vi "Open Gyro.vi"(8 "Gain":dbl=0.07, 9 "Analog Channel":T1=enum."AI 1", 11 "Gyro ID (1 or 2)":i32) -> ()   [LabVIEW 2015]
uses:
  <vilib>/Rock Robotics/SystemInterfaces/AI/FPGA_AIChannel.ctl
  Robot Global Data.vi
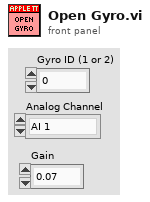
[diagram p1: front panel]
types:
  T1 = typedef "FPGA_AIChannel.ctl" = enum8{"AI 0", "AI 1", "AI 2", "AI 3", "AI MXP 0", "AI MXP 1", "AI MXP 2", "AI MXP 3", "Invalid"}
  T2 = typedef "WPI_AnalogChannelDevRef.ctl" = cluster{"DevStatus":errorcluster, "Analog Channel":T1}
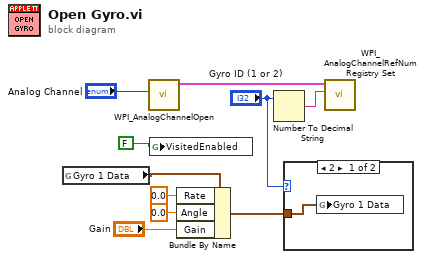
[diagram p0: block diagram]
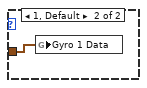
[diagram p2: hidden frame]
diagram:
  n1 = global read "Robot Global Data.vi" "Gyro 1 Data"() -> (w2:cluster{"Rate":dbl, "Angle":dbl, "Gain":dbl})
  n2 = call <vilib>:"WPI_AnalogChannelOpen.vi"("Analog Channel"="Analog Channel") -> ("AIDeviceRef"=w9:T2)  [unwired: 9 in, 1 out]
  n3 = global write "Robot Global Data.vi" "VisitedEnabled"(FALSE ("VisitedEnabled")) -> ()
  n4 = Bundle By Name(cluster=w2, "Rate"=0.0, "Angle"=0.0, "Gain"="Gain") -> (w3:cluster{"Rate":dbl, "Angle":dbl, "Gain":dbl})
  n5 = Number To Decimal String(number="Gyro ID (1 or 2)") -> (decimal integer string=w8:string)  [unwired: 1 in]
  n6 = case shown="2" "Gyro ID (1 or 2)" {
    tunnel: w3 -> [w11 w12]
    frame 2 {
      n7 = global write "Robot Global Data.vi" "Gyro 1 Data"(w11) -> ()
    }
    frame 1, Default {
      n8 = global write "Robot Global Data.vi" "Gyro 1 Data"(w12) -> ()
    }
  }
  n9 = call <vilib>:"WPI_AnalogChannelRefNum Registry Set.vi"("refnum name"=w8, "AIDeviceRef"=w9) -> ()  [unwired: 8 in, 2 out]
